vi "诊断标定4.vi"(8 "CAN端口":u16(ring), 9 "设备索引号":u16(ring), 10 "CAN卡类型":u32(ring)=4) -> ()   [LabVIEW 2013] (continued)
                                n469 = for {
                                N: 20 -> [_]
                                tunnel: [""] -> w840 mode=indexing
                                }
                                n470 = local read "从板个数"() -> (w842:dbl)
                                n471 = Increment(x=w842) -> (x+1=w838:dbl)
                                n472 = call "表格数据输入-8.6.vi"("行数"=w838, "列数"=u32 1, "字符串数组"=w840, "表格引用"=w841) -> ()  [unwired: 8 in]
                              }
                              frame "电压起始值" {
                                n473 = local read "从板个数"() -> (w846:dbl)
                                n474 = Increment(x=w846) -> (x+1=w845:dbl)
                                n475 = control-ref of="项目信息"() -> (w852:refnum<vi>)
                                n476 = for {
                                N: w845 -> [_]
                                tunnel: [""] -> w851 mode=indexing
                                }
                                n477 = Multiply(x=u8 1, y=w846) -> (x*y=w848:dbl)
                                n478 = Add(x=w848, y=u8 21) -> (x+y=w844:dbl)
                                n479 = call "表格数据输入-8.6.vi"("行数"=w844, "列数"=u32 1, "字符串数组"=w851, "表格引用"=w852) -> ()  [unwired: 8 in]
                              }
                              frame "温度个数" {
                                n480 = local read "从板个数"() -> (w856:dbl)
                                n481 = Increment(x=w856) -> (x+1=w855:dbl)
                                n482 = control-ref of="项目信息"() -> (w862:refnum<vi>)
                                n483 = for {
                                N: w855 -> [_]
                                tunnel: [""] -> w861 mode=indexing
                                }
                                n484 = Multiply(x=u8 2, y=w856) -> (x*y=w858:dbl)
                                n485 = Add(x=w858, y=u8 22) -> (x+y=w854:dbl)
                                n486 = call "表格数据输入-8.6.vi"("行数"=w854, "列数"=u32 1, "字符串数组"=w861, "表格引用"=w862) -> ()  [unwired: 8 in]
                              }
                              frame "温度起始值" {
                                n487 = local read "从板个数"() -> (w866:dbl)
                                n488 = Increment(x=w866) -> (x+1=w865:dbl)
                                n489 = control-ref of="项目信息"() -> (w872:refnum<vi>)
                                n490 = for {
                                N: w865 -> [_]
                                tunnel: [""] -> w871 mode=indexing
                                }
                                n491 = Multiply(x=u8 3, y=w866) -> (x*y=w868:dbl)
                                n492 = Add(x=w868, y=u8 23) -> (x+y=w864:dbl)
                                n493 = call "表格数据输入-8.6.vi"("行数"=w864, "列数"=u32 1, "字符串数组"=w871, "表格引用"=w872) -> ()  [unwired: 8 in]
                              }
                              frame "保险位置" {
                                n494 = local read "从板个数"() -> (w876:dbl)
                                n495 = control-ref of="项目信息"() -> (w882:refnum<vi>)
                                n496 = for {
                                N: 10 -> [_]
                                tunnel: [""] -> w881 mode=indexing
                                }
                                n497 = Multiply(x=u8 4, y=w876) -> (x*y=w878:dbl)
                                n498 = Add(x=w878, y=u8 24) -> (x+y=w875:dbl)
                                n499 = call "表格数据输入-8.6.vi"("行数"=w875, "列数"=u32 1, "字符串数组"=w881, "表格引用"=w882) -> ()  [unwired: 8 in]
                              }
                              frame "电池额定实际容量" {
                                w884 = 0.0 ("值")
                                n500 = control-ref of="电池实际容量(A)"() -> (w885:refnum<vi>)
                                n501 = control-ref of="电池额定容量(A)"() -> (w886:refnum<vi>)
                                n502 = property class="DigNum (严格)"(reference=w885, "Value"=w884) -> ()  [unwired: 1 in, 2 out]
                                n503 = property class="DigNum (严格)"(reference=w886, "Value"=w884) -> ()  [unwired: 1 in, 2 out]
                              }
                              frame "SOC" {
                                n504 = control-ref of="SOC(%)"() -> (w887:refnum<vi>)
                                n505 = property class="DigNum (严格)"(reference=w887, "Value"=0.0 ("值")) -> ()  [unwired: 1 in, 2 out]
                              }
                              frame "配置文件版本" {
                                n506 = control-ref of="配置文件版本"() -> (w889:refnum<vi>)
                                n507 = property class="Str"(reference=w889, "Value"="" ("值")) -> ()  [unwired: 1 in, 2 out]
                              }
                              frame "参数修改记录" {
                                n508 = control-ref of="使用者"() -> (w892:refnum<vi>)
                                n509 = control-ref of="系统时钟"() -> (w893:refnum<vi>)
                                n510 = property class="DigNum (严格)"(reference=w892, "Value"=0.0 ("值")) -> ()  [unwired: 1 in, 2 out]
                                n511 = property class="Str"(reference=w893, "Value"="" ("值")) -> ()  [unwired: 1 in, 2 out]
                              }
                              frame "校正时钟" {
                                n512 = control-ref of="系统时钟"() -> (w895:refnum<vi>)
                                n513 = property class="Str"(reference=w895, "Value"="" ("值")) -> ()  [unwired: 1 in, 2 out]
                              }
                              frame "车牌号" {
                                n514 = control-ref of="车架(牌)号"() -> (w897:refnum<vi>)
                                n515 = property class="Str"(reference=w897, "Value"="" ("值")) -> ()  [unwired: 1 in, 2 out]
                              }
                              frame "SOH" {
                                n516 = control-ref of="SOH(%)"() -> (w900:refnum<vi>)
                                n517 = property class="DigNum (严格)"(reference=w900, "Value"=0.0 ("值")) -> ()  [unwired: 1 in, 2 out]
                              }
                              frame "一级故障阀值" {
                                n518 = local write "一级故障"(T9 {"总电压过高"=0.0, "整组电压不均衡"=0.0, "SOC过高"=0.0, "单体电压过高"=0.0, "总电压过低"=0.0, "温度过高"=0.0, "温度过低"=0.0, "单组电压不均衡"=0.0, "整组温度不均衡"=0.0, "单组温度不均衡"=0.0, "单体电压过低"=0.0, "充电电流过高"=0.0, "放电电流过高"=0.0, "SOC过低"=0.0, "内阻过大"=0.0, "极柱温度过高"=0.0, "SOH过低"=0.0} ("一级故障")) -> ()
                              }
                              frame "二级故障阀值" {
                                n519 = local write "一级故障 2"(T9 {"总电压过高"=0.0, "整组电压不均衡"=0.0, "SOC过高"=0.0, "单体电压过高"=0.0, "总电压过低"=0.0, "温度过高"=0.0, "温度过低"=0.0, "单组电压不均衡"=0.0, "整组温度不均衡"=0.0, "单组温度不均衡"=0.0, "单体电压过低"=0.0, "充电电流过高"=0.0, "放电电流过高"=0.0, "SOC过低"=0.0, "内阻过大"=0.0, "极柱温度过高"=0.0, "SOH过低"=0.0} ("一级故障")) -> ()
                              }
                              frame "三级故障阀值" {
                                n520 = local write "一级故障 3"(T9 {"总电压过高"=0.0, "整组电压不均衡"=0.0, "SOC过高"=0.0, "单体电压过高"=0.0, "总电压过低"=0.0, "温度过高"=0.0, "温度过低"=0.0, "单组电压不均衡"=0.0, "整组温度不均衡"=0.0, "单组温度不均衡"=0.0, "单体电压过低"=0.0, "充电电流过高"=0.0, "放电电流过高"=0.0, "SOC过低"=0.0, "内阻过大"=0.0, "极柱温度过高"=0.0, "SOH过低"=0.0} ("一级故障")) -> ()
                              }
                              frame "加热控制参数" {
                                n521 = local write "加热控制参数"(T10 {"风机开启温度"=0.0, "风机关闭温度"=0.0, "加热开启温度"=0.0, "加热关闭温度"=0.0, "风机开启温差"=0.0, "风机关闭温差"=0.0, "加热关闭温差"=0.0} ("加热控制参数")) -> ()
                              }
                              frame "充电控制参数" {
                                n522 = local write "一级故障 5"(T11 {"最大允许单体电压"=0.0, "最大允许总电压"=0.0, "最小允许单体电压"=0.0, "最大允许充电电流"=0.0, "最小允许充电电流"=0.0, "最大允许充电温度"=0.0, "最小允许充电温度"=0.0, "电流步长"=0.0} ("一级故障 5")) -> ()
                              }
                              frame "电池信息1" {
                                w906 = ""
                                w907 = 0.0 ("电池串联")
                                n523 = local read "电池信息"() -> (w909:T12)
                                n524 = Bundle By Name(cluster=w909, "电池串联"=w907, "电池并联"=w907, "电池包额定容量"=w907, "电池包额定能量"=w907, "电池包额定总电压"=w907, "实际容量"=w907, "电池厂家"=w906, "电池类型"=w906, "电池生产日期"=w906) -> (w908:T12)
                                n525 = local write "电池信息"(w908) -> ()
                              }
                              frame "电池包组号" {
                                n526 = local read "电池信息"() -> (w912:T12)
                                n527 = Bundle By Name(cluster=w912, "电池包组号"="") -> (w911:T12)
                                n528 = local write "电池信息"(w911) -> ()
                              }
                              frame "充放电安时" {
                                w913 = 0.0 ("累计充电总安时")
                                n529 = local read "电池信息"() -> (w915:T12)
                                n530 = Bundle By Name(cluster=w915, "累计充电总安时"=w913, "累计放电总安时"=w913) -> (w914:T12)
                                n531 = local write "电池信息"(w914) -> ()
                              }
                              frame "电池充放电次数" {
                                w916 = 0.0 ("累计充电总安时")
                                n532 = local read "电池信息"() -> (w918:T12)
                                n533 = Bundle By Name(cluster=w918, "电池充满次数"=w916, "电池放空次数"=w916, "电池充电次数"=w916) -> (w917:T12)
                                n534 = local write "电池信息"(w917) -> ()
                              }
                            }
                          }
                          frame "从板" {
                            n535 = case shown="\"二级故障阀值\"" w919 {
                              frame "假", Default {
                              }
                              frame "电压起始值" {
                                n536 = control-ref of="项目信息 2"() -> (w920:refnum<vi>)
                                n537 = for {
                                N: 2 -> [_]
                                tunnel: [""] -> w924 mode=indexing
                                }
                                n538 = call "表格数据输入-8.6.vi"("行数"=u32 0, "列数"=u32 1, "字符串数组"=w924, "表格引用"=w920) -> ()  [unwired: 8 in]
                              }
                              frame "通道电压个数" {
                                n539 = control-ref of="项目信息 2"() -> (w926:refnum<vi>)
                                n540 = for {
                                N: 20 -> [_]
                                tunnel: [""] -> w930 mode=indexing
                                }
                                n541 = call "表格数据输入-8.6.vi"("行数"=u32 2, "列数"=u32 1, "字符串数组"=w930, "表格引用"=w926) -> ()  [unwired: 8 in]
                              }
                              frame "保险位置" {
                                n542 = control-ref of="项目信息 2"() -> (w932:refnum<vi>)
                                n543 = for {
                                N: 10 -> [_]
                                tunnel: [""] -> w936 mode=indexing
                                }
                                n544 = call "表格数据输入-8.6.vi"("行数"=u32 24, "列数"=u32 1, "字符串数组"=w936, "表格引用"=w932) -> ()  [unwired: 8 in]
                              }
                              frame "温度起始值" {
                                n545 = control-ref of="项目信息 2"() -> (w938:refnum<vi>)
                                n546 = for {
                                N: 2 -> [_]
                                tunnel: [""] -> w942 mode=indexing
                                }
                                n547 = call "表格数据输入-8.6.vi"("行数"=u32 22, "列数"=u32 1, "字符串数组"=w942, "表格引用"=w938) -> ()  [unwired: 8 in]
                              }
                              frame "加热控制参数" {
                                n548 = local write "加热控制参数"(T10 {"风机开启温度"=0.0, "风机关闭温度"=0.0, "加热开启温度"=0.0, "加热关闭温度"=0.0, "风机开启温差"=0.0, "风机关闭温差"=0.0, "加热关闭温差"=0.0} ("加热控制参数")) -> ()
                              }
                              frame "一级故障阀值" {
                                n549 = local write "一级故障 6"(T14 {"电压过高"=0.0, "电压过低"=0.0, "温度过高"=0.0, "温度过低"=0.0, "电压不均衡(V)"=0.0, "温度不均衡"=0.0, "SOC过低"=0.0} ("一级故障 6")) -> ()
                              }
                              frame "二级故障阀值" {
                                n550 = local write "一级故障 7"(T14 {"电压过高"=0.0, "电压过低"=0.0, "温度过高"=0.0, "温度过低"=0.0, "电压不均衡(V)"=0.0, "温度不均衡"=0.0, "SOC过低"=0.0} ("一级故障 7")) -> ()
                              }
                              frame "三级故障阀值" {
                                n551 = local write "一级故障 8"(T14 {"电压过高"=0.0, "电压过低"=0.0, "温度过高"=0.0, "温度过低"=0.0, "电压不均衡(V)"=0.0, "温度不均衡"=0.0, "SOC过低"=0.0} ("一级故障 7")) -> ()
                              }
                            }
                          }
                        }
                      }
                      frame #1 {
                        n552 = call <vilib>:"Set Busy.vi"("disable click? (T)"=FALSE) -> ()  [unwired: 3 in, 8 out]
                        n553 = global write "EV05全局变量1.vi" "写入超时"(FALSE ("写入超时")) -> ()
                        n554 = Wait Until Next ms Multiple(millisecond multiple=u32 20 ("毫秒倍数")) -> ()  [unwired: 1 out]
                        n555 = global write "EV05全局变量1.vi" "流控帧 2"(FALSE ("流控帧 2")) -> ()
                        n556 = local write "控制1"(TRUE ("控制1")) -> ()
                        n557 = local write "写?"(FALSE ("写?")) -> ()
                        n558 = local write "消除"(TRUE ("消除")) -> ()
                      }
                      frame #2 {
                        n559 = local read "设备索引号"() -> (w960:u16)
                        n560 = local read "CAN卡类型"() -> (w961:u32)
                        n561 = local read "CAN端口"() -> (w959:u16)
                        n562 = stacked-sequence {
                          tunnel: w961 -> [w964 w973]
                          tunnel: w960 -> [w963 w972]
                          tunnel: w959 -> [w962 w971]
                          tunnel: w958 -> [_ w970]
                          tunnel: w957 -> [_ w969]
                          tunnel: w956 -> [_ w968]
                          tunnel: w955 -> [_ w967]
                          frame #0 {
                            n563 = dll-call lib="PTH1Aabs EEV05EV05监控上位机-EV05EV05data\nusbcan.dll" fn="VCI_ClearBuffer"("DeviceType"=w964, "DeviceInd"=w963, "CANInd"=w962) -> (error out=w965:errorcluster)  [unwired: 4 in, 4 out]
                            n564 = call <vilib>:"Clear Errors.vi"("error in (no error)"=w965) -> ()  [unwired: 6 in, 1 out]
                          }
                          frame #1 {
                            n565 = call "多帧发送机制(EV05).vi"("can卡类型"=w973, "设备索引号"=w972, "CAN端口"=w971, "命令"=w969, "板号"=w968, "命令序号"=w970, "输入数据"=w967) -> ("错误输出"=w966:errorcluster)  [unwired: 1 in, 11 out]
                            n566 = call <vilib>:"Clear Errors.vi"("error in (no error)"=w966) -> ()  [unwired: 6 in, 1 out]
                          }
                        }
                        "命令序号" <- w958
                      }
                      frame #3 {
                        n567 = while {
                          tunnel: [w978] -> w975
                          tunnel: [w977] -> w974
                          i -> [w981]
                          stop <- w978 stop-if-true
                          n568 = local read "强制停止"() -> (w976:bool)
                          n569 = global read "EV05全局变量1.vi" "写入超时"() -> (w977:bool)
                          n570 = Greater Or Equal?(x=w981, y=25) -> (x >= y?=w979:bool)
                          n571 = Compound Arithmetic op=OR(w976, w977, w979) -> (w978:bool)
                          n572 = Wait Until Next ms Multiple(millisecond multiple=u32 100 ("毫秒倍数")) -> ()  [unwired: 1 out]
                        }
                      }
                      frame #4 {
                        n573 = call <vilib>:"Unset Busy.vi"() -> ()  [unwired: 11 in, 1 out]
                        n574 = case shown="假" w983 {
                          tunnel: w984 -> [w987 _]
                          frame False {
                            n575 = control-ref of="结果"() -> (w986:refnum<vi>)
                            n576 = Concatenate Strings(w987, "     读取失败" ("字符串")) -> (w989:string)
                            n577 = Build Array(w989) -> (w985:string[])
                            n578 = call "表格编辑.vi"("新元素/子数组"=w985, "活动单元格:单元格背景色"=u32 16740749, "MCListbox引用句柄"=w986) -> ()  [unwired: 9 out]
                          }
                          frame True {
                          }
                        }
                      }
                      frame #5 {
                        n579 = Increment(x=w993) -> (x+1=w992:i32)
                        n580 = Equal?(x=w994, y=w992) -> (x = y?=w991:bool)
                        n581 = case shown="真" w991 {
                          frame False {
                          }
                          frame True {
                            n582 = control-ref of="结果"() -> (w996:refnum<vi>)
                            n583 = Concatenate Strings("读取完成" ("字符串")) -> (w998:string)
                            n584 = Build Array(w998) -> (w995:string[])
                            n585 = call "表格编辑.vi"("新元素/子数组"=w995, "活动单元格:单元格背景色"=u32 21937, "MCListbox引用句柄"=w996) -> ()  [unwired: 9 out]
                          }
                        }
                      }
                    }
                  }
                }
              }
            }
            n586 = stacked-sequence {
              tunnel: w655 -> [_]
              frame #0 {
                n587 = local write "强制停止"(FALSE ("强制停止")) -> ()
              }
            }
          }
          frame "全部读取" {
            n588 = stacked-sequence {
              seq-local: [w1003 _ _] -> [_ _ w1489]
              seq-local: [w1002 _ _] -> [_ _ w1488]
              tunnel: [_ w1194 _] -> w1000
              frame #0 {
                n589 = local read "主从选择"() -> (w1003:enum32{"主板", "从板"})
                n590 = local read "路径"() -> (w1004:path)
                n591 = Empty String/Path?(string/path=w1004) -> (empty?=w1002:bool)
                n592 = disable-structure shown="禁用" {
                  disable-tunnel: w1004 -> [w1007 _]
                  disable-tunnel: w1002 -> [w1006 _]
                  disable-tunnel: w1003 -> [w1005 _]
                  frame Disabled {
                    n593 = case shown="假" w1006 {
                      tunnel: w1007 -> [w1011 _]
                      tunnel: w1005 -> [w1010 _]
                      frame False {
                        n594 = control-ref of="结果"() -> (w1008:refnum<vi>)
                        n595 = call-poly <vilib>:"Read From Spreadsheet File.vi"("file path (dialog if empty)"=w1011) -> ("all rows"=w1009:string[][])  [unwired: 3 in, 7 out]
                        n596 = case shown="\"主板\", 默认" w1010 {
                          tunnel: w1009 -> [w1013 w1108]
                          tunnel: w1008 -> [w1012 w1107]
                          frame "主板", Default {
                            n597 = stacked-sequence {
                              tunnel: w1013 -> [w1022 w1046 w1103]
                              tunnel: w1012 -> [w1019 _ w1074]
                              frame #0 {
                                n598 = Index Array(array=w1022, index (col)=3 ("禁用的索引 (列)")) -> (element=w1036:string[])  [unwired: 1 in]
                                n599 = Index Array(array=w1022, index (col)=1 ("禁用的索引 (列)")) -> (element=w1042:string[])  [unwired: 1 in]
                                n600 = Delete From Array(array=w1036, length=4 ("长度"), index=0 ("索引")) -> (deleted portion=w1033:string[], array with subset deleted=w1027:string[])
                                n601 = Delete From Array(array=w1042, length=1 ("长度"), index=0 ("索引")) -> (deleted portion=w1039:string[], array with subset deleted=w1016:string[])
                                n602 = Build Array("正在读取主板配置文件...") -> (w1020:string[])
                                n603 = Index Array(array=w1027) -> (element #1=w1026:string, element #2=w1025:string, element #3=w1024:string, element #4=w1023:string)  [unwired: 4 in]
                                n604 = for {
                                tunnel: w1033 -> [w1045] mode=indexing
                                tunnel: [w1044] -> w1032 mode=indexing
                                n605 = Fract/Exp String To Number(string=w1045) -> (number=w1044:dbl)  [unwired: 4 out]
                                }
                                n606 = Index Array(array=w1039) -> (element=w1038:string)  [unwired: 1 in]
                                n607 = global write "读配置文件全局.vi" "表格输入"(w1016) -> ()
                                n608 = call "表格编辑.vi"("新元素/子数组"=w1020, "活动单元格:单元格背景色"=u32 6618880, "MCListbox引用句柄"=w1019) -> ()  [unwired: 9 out]
                                n609 = Decimal String To Number(string=w1038) -> (number=w1017:i32)  [unwired: 1 in, 2 out]
                                n610 = global read "读配置文件全局.vi" "项目信息"() -> (w1015:T21)
                                n611 = Index Array(array=w1032) -> (element #1=w1031:dbl, element #2=w1030:dbl, element #3=w1029:dbl, element #4=w1028:dbl)  [unwired: 4 in]
                                n612 = global write "读配置文件全局.vi" "从板个数"(w1017) -> ()
                                n613 = Bundle(cluster=w1015, "电池额定容量"=w1031, "电池实际容量"=w1030, "车牌号"=w1026, "配置文件版本"=w1025, "SOH"=w1028, "SOC"=w1029, "产品编号"=w1024, "系统时钟"=w1023) -> (w1014:T21)  [unwired: 1 out]
                                n614 = global write "读配置文件全局.vi" "项目信息"(w1014) -> ()
                              }
                              frame #1 {
                                n615 = Index Array(array=w1046, index (col)=3 ("禁用的索引 (列)")) -> (element=w1064:string[])  [unwired: 1 in]
                                n616 = Index Array(array=w1046, index (col)=5 ("禁用的索引 (列)")) -> (element=w1058:string[])  [unwired: 1 in]
                                n617 = for {
                                tunnel: w1058 -> [w1071] mode=indexing
                                tunnel: [w1070] -> w1057 mode=indexing
                                n618 = Fract/Exp String To Number(string=w1071) -> (number=w1070:dbl)  [unwired: 4 out]
                                }
                                n619 = Delete From Array(array=w1064, length=17 ("长度"), index=8 ("索引")) -> (deleted portion=w1062:string[])  [unwired: 1 out]
                                n620 = for {
                                tunnel: w1062 -> [w1073] mode=indexing
                                tunnel: [w1072] -> w1060 mode=indexing
                                n621 = Fract/Exp String To Number(string=w1073) -> (number=w1072:dbl)  [unwired: 4 out]
                                }
                                n622 = global write "读配置文件全局.vi" "二级故障"(w1057) -> ()
                                n623 = global write "读配置文件全局.vi" "一级故障"(w1060) -> ()
                                n624 = Index Array(array=w1046, index (col)=7 ("禁用的索引 (列)")) -> (element=w1055:string[])  [unwired: 1 in]
                                n625 = Index Array(array=w1046, index (col)=9 ("禁用的索引 (列)")) -> (element=w1052:string[])  [unwired: 1 in]
                                n626 = for {
                                tunnel: w1055 -> [w1069] mode=indexing
                                tunnel: [w1068] -> w1054 mode=indexing
                                n627 = Fract/Exp String To Number(string=w1069) -> (number=w1068:dbl)  [unwired: 4 out]
                                }
                                n628 = for {
                                tunnel: w1052 -> [w1067] mode=indexing
                                tunnel: [w1066] -> w1051 mode=indexing
                                n629 = Fract/Exp String To Number(string=w1067) -> (number=w1066:dbl)  [unwired: 4 out]
                                }
                                n630 = Delete From Array(array=w1051, length=6 ("长度"), index=0 ("索引")) -> (deleted portion=w1048:dbl[], array with subset deleted=w1047:dbl[])
                                n631 = global write "读配置文件全局.vi" "三级故障"(w1054) -> ()
                                n632 = global write "读配置文件全局.vi" "加热控制参数"(w1048) -> ()
                                n633 = global write "读配置文件全局.vi" "充电控制参数"(w1047) -> ()
                              }
                              frame #2 {
                                n634 = call <vilib>:"Unset Busy.vi"() -> ()  [unwired: 2 in, 10 out]
                                n635 = Index Array(array=w1103, index (col)=11 ("禁用的索引 (列)")) -> (element=w1100:string[])  [unwired: 1 in]
                                n636 = Delete From Array(array=w1100, length=6 ("长度"), index=0 ("索引")) -> (deleted portion=w1082:string[], array with subset deleted=w1081:string[])
                                n637 = for {
                                tunnel: w1081 -> [w1106] mode=indexing
                                tunnel: [w1105] -> w1099 mode=indexing
                                n638 = Fract/Exp String To Number(string=w1106) -> (number=w1105:dbl)  [unwired: 4 out]
                                }
                                n639 = Index Array(array=w1082) -> (element #1=w1098:string, element #2=w1097:string, element #3=w1096:string, element #4=w1095:string, element #5=w1094:string, element #6=w1093:string)  [unwired: 6 in]
                                n640 = Index Array(array=w1099) -> (element #1=w1092:dbl, element #2=w1091:dbl, element #3=w1090:dbl, element #4=w1089:dbl, element #5=w1088:dbl, element #6=w1087:dbl, element #7=w1086:dbl, element #8=w1085:dbl, element #9=w1084:dbl, element #10=w1083:dbl, element #11=w1078:dbl)  [unwired: 11 in]
                                n641 = global read "读配置文件全局.vi" "电池信息"() -> (w1080:T12)
                                n642 = Build Array("配置文件读取完成") -> (w1076:string[])
                                n643 = Bundle(cluster=w1080, "电池串联"=w1092, "电池并联"=w1091, "累计放电总安时"=w1089, "电池包额定容量"=w1088, "电池包额定能量"=w1087, "电池包额定总电压"=w1086, "累计充电总安时"=w1090, "电池充满次数"=w1085, "电池放空次数"=w1084, "电池充电次数"=w1083, "电池生产日期"=w1098, "电池厂家"=w1097, "电池类型"=w1096, "电池包组号"=w1095, "电池包产权标识"=w1094, "电池应用车型"=w1093, "实际容量"=w1078) -> (w1079:T12)
                                n644 = call "表格编辑.vi"("新元素/子数组"=w1076, "活动单元格:单元格背景色"=u32 6618880, "MCListbox引用句柄"=w1074) -> ()  [unwired: 9 out]
                                n645 = global write "读配置文件全局.vi" "电池信息"(w1079) -> ()
                              }
                            }
                          }
                          frame "从板" {
                            n646 = stacked-sequence {
                              tunnel: w1108 -> [w1116 w1144 w1188]
                              tunnel: w1107 -> [w1113 _ w1164]
                              frame #0 {
                                n647 = Index Array(array=w1116, index (col)=1 ("禁用的索引 (列)")) -> (element=w1126:string[])  [unwired: 1 in]
                                n648 = Index Array(array=w1116, index (col)=3 ("禁用的索引 (列)")) -> (element=w1120:string[])  [unwired: 1 in]
                                n649 = Delete From Array(array=w1126, length=1 ("长度"), index=0 ("索引")) -> (deleted portion=w1123:string[], array with subset deleted=w1110:string[])
                                n650 = Delete From Array(array=w1120, length=6 ("长度"), index=0 ("索引")) -> (deleted portion=w1117:string[])  [unwired: 1 out]
                                n651 = for {
                                tunnel: w1117 -> [w1129] mode=indexing
                                tunnel: [w1128] -> w1109 mode=indexing
                                i -> [w1130]
                                n652 = Fract/Exp String To Number(string=w1129, default (0 dbl)=w1130) -> (number=w1128:i32)  [unwired: 3 out]
                                }
                                n653 = Index Array(array=w1123) -> (element=w1122:string)  [unwired: 1 in]
                                n654 = global write "读配置文件全局2.vi" "表格"(w1110) -> ()
                                n655 = Build Array("正在读取从板配置文件...") -> (w1114:string[])
                                n656 = Decimal String To Number(string=w1122) -> (number=w1111:i32)  [unwired: 1 in, 2 out]
                                n657 = call "表格编辑.vi"("新元素/子数组"=w1114, "活动单元格:单元格背景色"=u32 6618880, "MCListbox引用句柄"=w1113) -> ()  [unwired: 9 out]
                                n658 = global write "读配置文件全局2.vi" "加热控制参数"(w1109) -> ()
                                n659 = global write "读配置文件全局2.vi" "从板板号"(w1111) -> ()
                              }
                              frame #1 {
                                n660 = Index Array(array=w1144, index (col)=3 ("禁用的索引 (列)")) -> (element=w1134:string[])  [unwired: 1 in]
                                n661 = Array Subset(array=w1134, index=6 ("索引"), length=7 ("长度")) -> (w1141:string[])
                                n662 = Array Subset(array=w1134, index=13 ("索引"), length=7 ("长度")) -> (w1140:string[])
                                n663 = Array Subset(array=w1134, index=20 ("索引"), length=7 ("长度")) -> (w1135:string[])
                                n664 = for {
                                tunnel: w1141 -> [w1151] mode=indexing
                                tunnel: [w1150] -> w1131 mode=indexing
                                n665 = Fract/Exp String To Number(string=w1151) -> (number=w1150:dbl)  [unwired: 4 out]
                                }
                                n666 = for {
                                tunnel: w1140 -> [w1149] mode=indexing
                                tunnel: [w1148] -> w1132 mode=indexing
                                n667 = Fract/Exp String To Number(string=w1149) -> (number=w1148:dbl)  [unwired: 4 out]
                                }
                                n668 = for {
                                tunnel: w1135 -> [w1147] mode=indexing
                                tunnel: [w1146] -> w1133 mode=indexing
                                n669 = Fract/Exp String To Number(string=w1147) -> (number=w1146:dbl)  [unwired: 4 out]
                                }
                                n670 = global write "读配置文件全局2.vi" "一级故障阀值"(w1131) -> ()
                                n671 = global write "读配置文件全局2.vi" "二级故障阀值"(w1132) -> ()
                                n672 = global write "读配置文件全局2.vi" "三级故障阀值"(w1133) -> ()
                              }
                              frame #2 {
                                n673 = Index Array(array=w1188, index (col)=5 ("禁用的索引 (列)")) -> (element=w1186:string[])  [unwired: 1 in]
                                n674 = Delete From Array(array=w1186, length=1 ("长度"), index=16 ("索引")) -> (deleted portion=w1182:string[], array with subset deleted=w1183:string[])
                                n675 = for {
                                tunnel: w1183 -> [w1191] mode=indexing
                                tunnel: [w1190] -> w1187 mode=indexing
                                n676 = Fract/Exp String To Number(string=w1191) -> (number=w1190:dbl)  [unwired: 4 out]
                                }
                                n677 = Index Array(array=w1187) -> (element #1=w1181:dbl, element #2=w1180:dbl, element #3=w1179:dbl, element #4=w1178:dbl, element #5=w1177:dbl, element #6=w1176:dbl, element #7=w1175:dbl, element #8=w1174:dbl, element #9=w1173:dbl, element #10=w1172:dbl, element #11=w1171:dbl, element #12=w1162:dbl, element #13=w1170:dbl, element #14=w1169:dbl, element #15=w1168:dbl, element #16=w1167:dbl, element #17=w1160:dbl, element #18=w1159:dbl, element #19=w1158:dbl, element #20=w1157:dbl, element #21=w1156:dbl, element #22=w1155:dbl)  [unwired: 22 in]
                                n678 = Build Array("配置文件读取完成") -> (w1165:string[])
                                n679 = Index Array(array=w1182, index=22 ("索引")) -> (element=w1161:string)
                                n680 = global read "读配置文件全局2.vi" "电池组信息"() -> (w1153:T15)
                                n681 = call "表格编辑.vi"("新元素/子数组"=w1165, "活动单元格:单元格背景色"=u32 6618880, "MCListbox引用句柄"=w1164) -> ()  [unwired: 9 out]
                                n682 = Bundle(cluster=w1153, "电池类型"=w1181, "电池厂家"=w1180, "电池地区"=w1179, "电池组序号"=w1178, "电池包串联数"=w1177, "电池包并联数"=w1176, "电池包安时数"=w1175, "电池包序号"=w1174, "充电次数"=w1173, "充满电时间"=w1172, "放空时间"=w1171, "车牌号"=w1161, "最大允许单体电压"=w1162, "最大允许总电压"=w1170, "最大允许温度"=w1169, "最小允许温度"=w1168, "最大允许充电电流"=w1167, "最小允许充电电流"=w1160, "最小允许单体电压"=w1159, "电流步长"=w1158, "SOC"=w1157, "充电总安时"=w1156, "放电总这时"=w1155) -> (w1152:T15)
                                n683 = call <vilib>:"Unset Busy.vi"() -> ()  [unwired: 2 in, 10 out]
                                n684 = global write "读配置文件全局2.vi" "电池组信息"(w1152) -> ()
                              }
                            }
                          }
                        }
                      }
                      frame True {
                      }
                    }
                  }
                  frame Enabled {
                  }
                }
                n685 = case shown="\"从板\"" w1003 {
                  frame "主板", Default {
                    w1192 = FALSE
                    n686 = global write "读配置文件全局.vi" "SOC判定"(w1192) -> ()
                    n687 = global write "读配置文件全局.vi" "SOH判定"(w1192) -> ()
                    n688 = global write "读配置文件全局.vi" "车牌号判定"(w1192) -> ()
                    n689 = global write "读配置文件全局.vi" "充放电安时判定"(w1192) -> ()
                    n690 = global write "读配置文件全局.vi" "电池包组号判定"(w1192) -> ()
                    n691 = global write "读配置文件全局.vi" "电池充放电次数判定"(w1192) -> ()
                    n692 = global write "读配置文件全局.vi" "电池信息1判定"(w1192) -> ()
                    n693 = global write "读配置文件全局.vi" "电压起始值判定"(w1192) -> ()
                    n694 = global write "读配置文件全局.vi" "通道电压数判定"(w1192) -> ()
                    n695 = global write "读配置文件全局.vi" "温度起始值判定"(w1192) -> ()
                    n696 = global write "读配置文件全局.vi" "保险位置判定"(w1192) -> ()
                    n697 = global write "读配置文件全局.vi" "产品编号判定"(w1192) -> ()
                    n698 = global write "读配置文件全局.vi" "充电控制参数判定"(w1192) -> ()
                    n699 = global write "读配置文件全局.vi" "从板个数判定"(w1192) -> ()
                    n700 = global write "读配置文件全局.vi" "电池额定实际容量判定"(w1192) -> ()
                    n701 = global write "读配置文件全局.vi" "电压个数判定"(w1192) -> ()
                    n702 = global write "读配置文件全局.vi" "二级故障判定"(w1192) -> ()
                    n703 = global write "读配置文件全局.vi" "加热控制参数判定"(w1192) -> ()
                    n704 = global write "读配置文件全局.vi" "配置文件版本判定"(w1192) -> ()
                    n705 = global write "读配置文件全局.vi" "三级故障判定"(w1192) -> ()
                    n706 = global write "读配置文件全局.vi" "温度个数判定"(w1192) -> ()
                    n707 = global write "读配置文件全局.vi" "一级故障判定"(w1192) -> ()
                  }
                  frame "从板" {
                    w1193 = FALSE
                    n708 = disable-structure shown="禁用" {
                      frame Disabled {
                        n709 = global read "读配置文件全局2.vi" "充电次数时间判定"() -> ()  [unwired: 1 in]
                        n710 = global read "读配置文件全局2.vi" "电池包信息1判定"() -> ()  [unwired: 1 in]
                        n711 = global read "读配置文件全局2.vi" "电池包序号判定"() -> ()  [unwired: 1 in]
                        n712 = global read "读配置文件全局2.vi" "充放电安时判定"() -> ()  [unwired: 1 in]
                        n713 = global read "读配置文件全局2.vi" "车牌号判定"() -> ()  [unwired: 1 in]
                        n714 = global read "读配置文件全局2.vi" "充电参数判定"() -> ()  [unwired: 1 in]
                        n715 = global read "读配置文件全局2.vi" "保险位置判定"() -> ()  [unwired: 1 in]
                      }
                      frame Enabled {
                      }
                    }
                    n716 = global write "读配置文件全局2.vi" "从板号判定"(w1193) -> ()
                    n717 = global write "读配置文件全局2.vi" "电压起始值判定"(w1193) -> ()
                    n718 = global write "读配置文件全局2.vi" "通道电压判定"(w1193) -> ()
                    n719 = global write "读配置文件全局2.vi" "保险位置判定"(w1193) -> ()
                    n720 = global write "读配置文件全局2.vi" "温度起始值判定"(w1193) -> ()
                    n721 = global write "读配置文件全局2.vi" "二级故障判定"(w1193) -> ()
                    n722 = global write "读配置文件全局2.vi" "三级故障判定"(w1193) -> ()
                    n723 = global write "读配置文件全局2.vi" "一级故障判定"(w1193) -> ()
                  }
                }
              }
              frame #1 {
                # "去掉加热控制信息 20140106"
                n724 = local read "主从选择"() -> (w1197:enum32{"主板", "从板"})
                n725 = case shown="\"主板\", 默认" w1197 {
                  tunnel: [string[] ["项目信息", "一级故障阀值", "二级故障阀值", "三级故障阀值", "加热控制信息", "充电控制信息", "电池信息"] string[] ["从板信息", "一级故障阀值", "二级故障阀值", "三级故障阀值"]] -> w1196
                  frame "主板", Default {
                  }
                  frame "从板" {
                  }
                }
                n726 = Array Size(array=w1196) -> (size(s)=w1195:i32)
                n727 = for {
                  tunnel: w1196 -> [w1213] mode=indexing
                  tunnel: w1197 -> [w1201]
                  tunnel: w1195 -> [w1205]
                  tunnel: [w1200] -> w1194
                  i -> [w1202]
                  n728 = case shown="\"主板\", 默认" w1201 {
                    tunnel: [w1443 w1471] -> w1207
                    tunnel: [w1442 w1472] -> w1208
                    tunnel: w1213 -> [w1439 w1468]
                    tunnel: [u8 0 ("板号") w1469] -> w1212
                    tunnel: [u8 0 ("板号") u8 0 ("板号")] -> w1211
                    tunnel: [w1438 w1467] -> w1209
                    frame "主板", Default {
                      n729 = case shown="\"历史信息\"" w1439 {
                        tunnel: [_ u8[] [1, 2, 3, 4, 5, 6, 13, 8, 7, 9, 10, 11, 12] u8[] [1] u8[] [2] u8[] [3] u8[] [1] u8[] [2] u8[] [1, 2, 3] u8[] [1, 2, 3, 4]] -> w1443
                        tunnel: [_ u8 128 ("命令") u8 129 ("命令") u8 129 ("命令") u8 129 ("命令") u8 130 ("命令") u8 130 ("命令") u8 131 ("命令") u8 132 ("命令")] -> w1442
                        tunnel: [_ string[] ["产品编号", "电压个数", "通道电压数", "电压起始值", "温度个数", "温度起始值", "保险位置", "电池额定实际容量", "SOC", "配置文件版本", "参数修改记录", "车牌号", "SOH"] string[] ["一级故障阀值"] string[] ["二级故障阀值"] string[] ["三级故障阀值"] string[] ["加热控制参数"] string[] ["充电控制参数"] _ string[] ["电池信息1", "电池包组号", "充放电安时", "电池充放电次数"]] -> w1438
                        frame "假", Default {
                        }
                        frame "项目信息" {
                        }
                        frame "一级故障阀值" {
                        }
                        frame "二级故障阀值" {
                        }
                        frame "三级故障阀值" {
                        }
                        frame "加热控制信息" {
                        }
                        frame "充电控制信息" {
                        }
                        frame "历史信息" {
                        }
                        frame "电池信息" {
                        }
                      }
                    }
                    frame "从板" {
                      n730 = case shown="\"从板信息\"" w1468 {
                        tunnel: [_ u8 0 ("命令") u8 2 ("命令") u8 2 ("命令") u8 2 ("命令") u8 3 ("命令")] -> w1472
                        tunnel: [_ u8[] [6, 1, 2, 3, 4, 5] u8[] [1] u8[] [2] u8[] [3] u8[] [1, 2, 3, 4, 5, 6, 7]] -> w1471
                        tunnel: [_ string[] ["从板号", "电压起始值", "通道电压节数", "保险位置", "温度起始值", "加热控制参数"] string[] ["一级故障阀值"] string[] ["二级故障阀值"] string[] ["三级故障阀值"] string[] ["电池包信息1", "电池包序号", "充放电安时", "充电次数时间", "SOC", "车牌号", "充电参数"]] -> w1467
                        frame "假", Default {
                        }
                        frame "从板信息" {
                        }
                        frame "一级故障阀值" {
                        }
                        frame "二级故障阀值" {
                        }
                        frame "三级故障阀值" {
                        }
                        frame "快换参数" {
                        }
                      }
                      n731 = local read "从板板号"() -> (w1469:u8)
                    }
                  }
                  n732 = Increment(x=w1202) -> (x+1=w1204:i32)
                  n733 = Equal?(x=w1205, y=w1204) -> (x = y?=w1203:bool)
                  n734 = case shown="\"从板\"" w1201 {
                    tunnel: w1202 -> [w1411 w1425]
                    frame "主板", Default {
                      n735 = case shown="0, 默认" w1411 {
                        tunnel: [T7."项目信息" ("主从板") T7."一级故障阀值" ("主从板") T7."二级故障阀值" ("主从板") T7."三级故障阀值" ("主从板") T7."控制参数" ("主从板") T7."电池信息" ("主从板")] -> w1410
                        frame 0, Default {
                          n736 = local write "1"(TRUE ("1")) -> ()
                        }
                        frame 1 {
                          n737 = local write "1 2"(TRUE ("1 2")) -> ()
                        }
                        frame 2 {
                          n738 = local write "1 3"(TRUE ("1 3")) -> ()
                        }
                        frame 3 {
                          n739 = local write "1 4"(TRUE ("1 4")) -> ()
                        }
                        frame 4, 5 {
                          n740 = local write "1 5"(TRUE ("1 5")) -> ()
                        }
                        frame 6 {
                          n741 = local write "1 11"(TRUE ("1 11")) -> ()
                        }
                      }
                      n742 = local write "主板2"(w1410) -> ()
                    }
                    frame "从板" {
                      n743 = case shown="4" w1425 {
                        tunnel: [T13."从板信息" ("等级 2") T13."从板信息" ("等级 2") T13."一级故障阀值" ("等级 2") T13."二级故障阀值" ("等级 2") T13."三级故障阀值" ("等级 2") T13."快换参数" ("等级 2")] -> w1424
                        frame 99, Default {
                          n744 = local write "1 6"(TRUE ("1 6")) -> ()
                        }
                        frame 0 {
                          n745 = local write "1 6"(TRUE ("1 6")) -> ()
                        }
                        frame 1 {
                          n746 = local write "1 7"(TRUE ("1 7")) -> ()
                        }
                        frame 2 {
                          n747 = local write "1 8"(TRUE ("1 8")) -> ()
                        }
                        frame 3 {
                          n748 = local write "1 9"(TRUE ("1 9")) -> ()
                        }
                        frame 4 {
                          n749 = local write "1 10"(TRUE ("1 10")) -> ()
                        }
                      }
                      n750 = local write "等级 2"(w1424) -> ()
                    }
                  }
                  n751 = Array Size(array=w1207) -> (size(s)=w1206:i32)
                  n752 = local write "命令"(w1208) -> ()
                  n753 = Build Array(w1211) -> (w1210:u8[])
                  n754 = while {
                    tunnel: w1207 -> [w1225] mode=indexing
                    tunnel: w1208 -> [w1226]
                    tunnel: w1212 -> [w1224]
                    tunnel: w1210 -> [w1223]
                    tunnel: w1209 -> [w1222] mode=indexing
                    tunnel: w1206 -> [w1218]
                    tunnel: w1203 -> [w1221]
                    tunnel: w1201 -> [w1215]
                    tunnel: [w1214] -> w1200
                    i -> [w1219]
                    stop <- w1214 stop-if-true
                    n755 = Increment(x=w1219) -> (x+1=w1220:i32)
                    n756 = Equal?(x=w1218, y=w1220) -> (x = y?=w1216:bool)
                    n757 = while {
                      tunnel: w1226 -> [w1235]
                      tunnel: w1225 -> [w1234]
                      tunnel: w1224 -> [w1233]
                      tunnel: w1223 -> [w1232]
                      tunnel: w1222 -> [w1230]
                      tunnel: w1221 -> [w1229]
                      tunnel: w1216 -> [w1228]
                      tunnel: w1215 -> [w1227]
                      stop <- w1231 stop-if-true
                      n758 = stacked-sequence {
                        seq-local: [_ _ _ w1384 _ _] -> [_ _ _ _ w1394 _]
                        tunnel: w1235 -> [_ _ w1372 _ _ _]
                        tunnel: w1234 -> [_ _ w1371 _ _ _]
                        tunnel: w1233 -> [_ _ w1370 _ _ _]
                        tunnel: w1232 -> [_ _ w1369 _ _ _]
                        tunnel: [_ _ _ w1385 _ _] -> w1231
                        tunnel: w1230 -> [w1237 _ _ _ w1393 _]
                        tunnel: w1229 -> [_ _ _ _ _ w1403]
                        tunnel: w1228 -> [_ _ _ _ _ w1401]
                        tunnel: w1227 -> [w1236 _ _ _ _ _]
                        frame #0 {
                          n759 = case shown="\"从板\"" w1236 {
                            tunnel: w1237 -> [w1238 w1330]
                            frame "主板", Default {
                              n760 = case shown="\"参数修改记录\"" w1238 {
                                frame "假", Default {
                                }
                                frame "产品编号" {
                                n761 = control-ref of="产品编号"() -> (w1240:refnum<vi>)
                                n762 = property class="Str"(reference=w1240, "Value"="") -> ()  [unwired: 1 in, 2 out]
                                }
                                frame "电压个数" {
                                n763 = local read "从板个数"() -> (w1246:dbl)
                                n764 = control-ref of="项目信息"() -> (w1244:refnum<vi>)
                                n765 = Increment(x=w1246) -> (x+1=w1245:dbl)
                                n766 = for {
                                N: w1245 -> [_]
                                tunnel: [""] -> w1243 mode=indexing
                                }
                                n767 = call "表格数据输入-8.6.vi"("行数"=u32 0, "列数"=u32 1, "字符串数组"=w1243, "表格引用"=w1244) -> ()  [unwired: 8 in]
                                }
                                frame "通道电压数" {
                                n768 = control-ref of="项目信息"() -> (w1252:refnum<vi>)
                                n769 = for {
                                N: 20 -> [_]
                                tunnel: [""] -> w1251 mode=indexing
                                }
                                n770 = local read "从板个数"() -> (w1253:dbl)
                                n771 = Increment(x=w1253) -> (x+1=w1249:dbl)
                                n772 = call "表格数据输入-8.6.vi"("行数"=w1249, "列数"=u32 1, "字符串数组"=w1251, "表格引用"=w1252) -> ()  [unwired: 8 in]
                                }
                                frame "电压起始值" {
                                n773 = local read "从板个数"() -> (w1257:dbl)
                                n774 = Increment(x=w1257) -> (x+1=w1256:dbl)
                                n775 = control-ref of="项目信息"() -> (w1263:refnum<vi>)
                                n776 = for {
                                N: w1256 -> [_]
                                tunnel: [""] -> w1262 mode=indexing
                                }
                                n777 = Multiply(x=u8 1, y=w1257) -> (x*y=w1259:dbl)
                                n778 = Add(x=w1259, y=u8 21) -> (x+y=w1255:dbl)
                                n779 = call "表格数据输入-8.6.vi"("行数"=w1255, "列数"=u32 1, "字符串数组"=w1262, "表格引用"=w1263) -> ()  [unwired: 8 in]
                                }
                                frame "温度个数" {
                                n780 = local read "从板个数"() -> (w1267:dbl)
                                n781 = Increment(x=w1267) -> (x+1=w1266:dbl)
                                n782 = control-ref of="项目信息"() -> (w1273:refnum<vi>)
                                n783 = for {
                                N: w1266 -> [_]
                                tunnel: [""] -> w1272 mode=indexing
                                }
                                n784 = Multiply(x=u8 2, y=w1267) -> (x*y=w1269:dbl)
                                n785 = Add(x=w1269, y=u8 22) -> (x+y=w1265:dbl)
                                n786 = call "表格数据输入-8.6.vi"("行数"=w1265, "列数"=u32 1, "字符串数组"=w1272, "表格引用"=w1273) -> ()  [unwired: 8 in]
                                }
                                frame "温度起始值" {
                                n787 = local read "从板个数"() -> (w1277:dbl)
                                n788 = Increment(x=w1277) -> (x+1=w1276:dbl)
                                n789 = control-ref of="项目信息"() -> (w1283:refnum<vi>)
                                n790 = for {
                                N: w1276 -> [_]
                                tunnel: [""] -> w1282 mode=indexing
                                }
                                n791 = Multiply(x=u8 3, y=w1277) -> (x*y=w1279:dbl)
                                n792 = Add(x=w1279, y=u8 23) -> (x+y=w1275:dbl)
                                n793 = call "表格数据输入-8.6.vi"("行数"=w1275, "列数"=u32 1, "字符串数组"=w1282, "表格引用"=w1283) -> ()  [unwired: 8 in]
                                }
                                frame "保险位置" {
                                n794 = local read "从板个数"() -> (w1287:dbl)
                                n795 = control-ref of="项目信息"() -> (w1293:refnum<vi>)
                                n796 = for {
                                N: 10 -> [_]
                                tunnel: [""] -> w1292 mode=indexing
                                }
                                n797 = Multiply(x=u8 4, y=w1287) -> (x*y=w1289:dbl)
                                n798 = Add(x=w1289, y=u8 24) -> (x+y=w1286:dbl)
                                n799 = call "表格数据输入-8.6.vi"("行数"=w1286, "列数"=u32 1, "字符串数组"=w1292, "表格引用"=w1293) -> ()  [unwired: 8 in]
                                }
                                frame "电池额定实际容量" {
                                w1295 = 0.0 ("值")
                                n800 = control-ref of="电池实际容量(A)"() -> (w1296:refnum<vi>)
                                n801 = control-ref of="电池额定容量(A)"() -> (w1297:refnum<vi>)
                                n802 = property class="DigNum (严格)"(reference=w1296, "Value"=w1295) -> ()  [unwired: 1 in, 2 out]
                                n803 = property class="DigNum (严格)"(reference=w1297, "Value"=w1295) -> ()  [unwired: 1 in, 2 out]
                                }
                                frame "SOC" {
                                n804 = control-ref of="SOC(%)"() -> (w1298:refnum<vi>)
                                n805 = property class="DigNum (严格)"(reference=w1298, "Value"=0.0 ("值")) -> ()  [unwired: 1 in, 2 out]
                                }
                                frame "配置文件版本" {
                                n806 = control-ref of="配置文件版本"() -> (w1300:refnum<vi>)
                                n807 = property class="Str"(reference=w1300, "Value"="" ("值")) -> ()  [unwired: 1 in, 2 out]
                                }
                                frame "参数修改记录" {
                                n808 = control-ref of="使用者"() -> (w1303:refnum<vi>)
                                n809 = control-ref of="系统时钟"() -> (w1304:refnum<vi>)
                                n810 = property class="DigNum (严格)"(reference=w1303, "Value"=0.0 ("值")) -> ()  [unwired: 1 in, 2 out]
                                n811 = property class="Str"(reference=w1304, "Value"="" ("值")) -> ()  [unwired: 1 in, 2 out]
                                }
                                frame "校正时钟" {
                                n812 = control-ref of="系统时钟"() -> (w1306:refnum<vi>)
                                n813 = property class="Str"(reference=w1306, "Value"="" ("值")) -> ()  [unwired: 1 in, 2 out]
                                }
                                frame "车牌号" {
                                n814 = control-ref of="车架(牌)号"() -> (w1308:refnum<vi>)
                                n815 = property class="Str"(reference=w1308, "Value"="" ("值")) -> ()  [unwired: 1 in, 2 out]
                                }
                                frame "SOH" {
                                n816 = control-ref of="SOH(%)"() -> (w1311:refnum<vi>)
                                n817 = property class="DigNum (严格)"(reference=w1311, "Value"=0.0 ("值")) -> ()  [unwired: 1 in, 2 out]
                                }
                                frame "一级故障阀值" {
                                n818 = local write "一级故障"(T9 {"总电压过高"=0.0, "整组电压不均衡"=0.0, "SOC过高"=0.0, "单体电压过高"=0.0, "总电压过低"=0.0, "温度过高"=0.0, "温度过低"=0.0, "单组电压不均衡"=0.0, "整组温度不均衡"=0.0, "单组温度不均衡"=0.0, "单体电压过低"=0.0, "充电电流过高"=0.0, "放电电流过高"=0.0, "SOC过低"=0.0, "内阻过大"=0.0, "极柱温度过高"=0.0, "SOH过低"=0.0} ("一级故障")) -> ()
                                }
                                frame "二级故障阀值" {
                                n819 = local write "一级故障 2"(T9 {"总电压过高"=0.0, "整组电压不均衡"=0.0, "SOC过高"=0.0, "单体电压过高"=0.0, "总电压过低"=0.0, "温度过高"=0.0, "温度过低"=0.0, "单组电压不均衡"=0.0, "整组温度不均衡"=0.0, "单组温度不均衡"=0.0, "单体电压过低"=0.0, "充电电流过高"=0.0, "放电电流过高"=0.0, "SOC过低"=0.0, "内阻过大"=0.0, "极柱温度过高"=0.0, "SOH过低"=0.0} ("一级故障")) -> ()
                                }
                                frame "三级故障阀值" {
                                n820 = local write "一级故障 3"(T9 {"总电压过高"=0.0, "整组电压不均衡"=0.0, "SOC过高"=0.0, "单体电压过高"=0.0, "总电压过低"=0.0, "温度过高"=0.0, "温度过低"=0.0, "单组电压不均衡"=0.0, "整组温度不均衡"=0.0, "单组温度不均衡"=0.0, "单体电压过低"=0.0, "充电电流过高"=0.0, "放电电流过高"=0.0, "SOC过低"=0.0, "内阻过大"=0.0, "极柱温度过高"=0.0, "SOH过低"=0.0} ("一级故障")) -> ()
                                }
                                frame "加热控制参数" {
                                n821 = local write "加热控制参数"(T10 {"风机开启温度"=0.0, "风机关闭温度"=0.0, "加热开启温度"=0.0, "加热关闭温度"=0.0, "风机开启温差"=0.0, "风机关闭温差"=0.0, "加热关闭温差"=0.0} ("加热控制参数")) -> ()
                                }
                                frame "充电控制参数" {
                                n822 = local write "一级故障 5"(T11 {"最大允许单体电压"=0.0, "最大允许总电压"=0.0, "最小允许单体电压"=0.0, "最大允许充电电流"=0.0, "最小允许充电电流"=0.0, "最大允许充电温度"=0.0, "最小允许充电温度"=0.0, "电流步长"=0.0} ("一级故障 5")) -> ()
                                }
                                frame "电池信息1" {
                                w1317 = ""
                                w1318 = 0.0 ("电池串联")
                                n823 = local read "电池信息"() -> (w1320:T12)
